vi "worksheet set landscape.vi"(8 "error in (no error)":errorcluster, 11 "worksheet":u32) -> (0 "error out":errorcluster)   [LabVIEW 8.6]
doc: "void worksheet_set_landscape(lxw_worksheet worksheet);"
uses:
  pending_lvxlsxwriter/xlsxwriter.dll
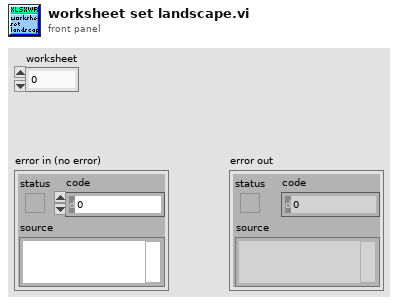
[diagram p1: front panel]
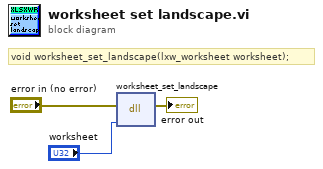
[diagram p0: block diagram]
diagram:
  # "void worksheet_set_landscape(lxw_worksheet worksheet);"
  n1 = dll-call lib="C:/Users/WDAGUtilityAccount/Desktop/pending_lvxlsxwriter/xlsxwriter.*" fn="worksheet_set_landscape"(error in="error in (no error)", "worksheet"="worksheet") -> (error out=→"error out":errorcluster)  [unwired: 4 in, 1 out]
